vi "String Scroll.vi"(11 "fp string refnum in":refnum<vi>) -> ()   [LabVIEW 2012]
doc: "SciScan 1.2 160622"
uses:
  <vilib>/Utility/inputDevices.llb/closeMouse.vi
  <vilib>/Utility/inputDevices.llb/mouseAcquire.vi
panel:
  in  "Error In":errorcluster
  out "Error Out":errorcluster
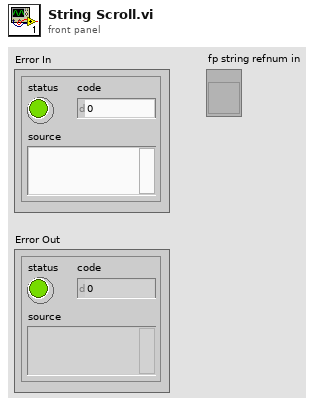
[diagram p1: front panel]
types:
  T1 = cluster{"Horizontal":i32, "Vertical":i32, "Scrolling":i32}
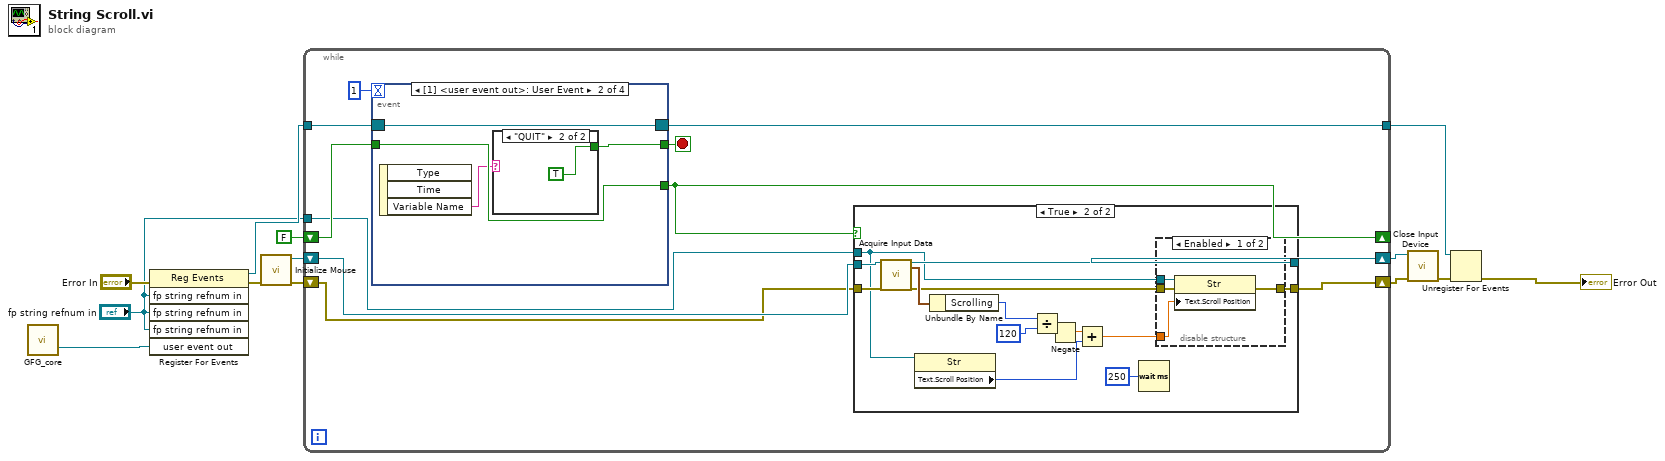
[diagram p0: block diagram]
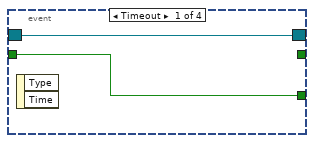
[diagram p2: hidden frame]
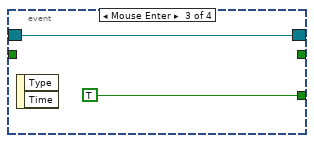
[diagram p4: hidden frame]
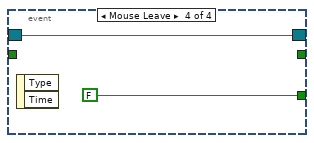
[diagram p5: hidden frame]
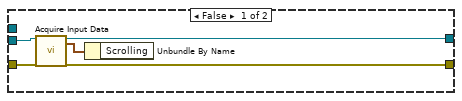
[diagram p6: hidden frame]
diagram:
  n1 = call "GFG_core.vi"() -> ("user event out"=w2:refnum<user-event>)  [unwired: 13 in, 6 out]
  n2 = register-events(error in="Error In", "fp string refnum in", "fp string refnum in", "fp string refnum in", w2) -> (reference out=w10:refnum<event-registration>, error out=w11:errorcluster)  [unwired: 1 in]
  n3 = call <vilib>:"Initialize Mouse.vi"("error in (no error)"=w11) -> ("error out"=w4:errorcluster, "device ID"=w3:refnum<k1>)  [unwired: 9 in]
  n4 = while {
    shift-right: [w21] -> w6
    shift-left: w4 -> [w23]
    shift-right: [w22] -> w5
    shift-left: w3 -> [w24]
    shift-right: [w19] -> _
    shift-left: FALSE -> [w18]
    tunnel: [w17] -> w7
    tunnel: "fp string refnum in" -> [w16]
    tunnel: w10 -> [w15]
    stop <- w14 stop-if-true
    n5 = event shown="[1] <user event out>: User Event" {
      selector: w15 -> [w25 w28 w32 w34]
      dyn-events: [w25 w28 w32 w34] -> w17
      timeout: 1 -> [_ _ _ _]
      tunnel: [w26 w29 TRUE FALSE] -> w19
      tunnel: w18 -> [w26 w29 _ _]
      tunnel: [_ w30 _ _] -> w14
      event Timeout {
        n6 = event-data() -> ()  [unwired: 1 in, 2 out]
      }
      event User Event {
        n7 = event-data() -> ("Variable Name"=w27:string)  [unwired: 1 in, 2 out]
        n8 = case shown="\"QUIT\"" w27 {
          tunnel: [_ TRUE] -> w30
          frame "False", Default {
          }
          frame "QUIT" {
          }
        }
      }
      event Mouse Enter {
        n9 = event-data() -> ()  [unwired: 1 in, 2 out]
      }
      event Mouse Leave {
        n10 = event-data() -> ()  [unwired: 1 in, 2 out]
      }
    }
    n11 = case shown="True" w19 {
      tunnel: w24 -> [w39 w54]
      tunnel: w23 -> [w40 w53]
      tunnel: [w38 w52] -> w22
      tunnel: [w37 w49] -> w21
      tunnel: w16 -> [_ w46]
      frame False {
        n12 = call-poly <vilib>:"Acquire Input Data.vi"("device ID"=w39, "error in (no error)"=w40) -> ("device ID"=w38:refnum<k1>, "axis info"=w36:T1, "error out"=w37:errorcluster)  [unwired: 14 in, 1 out]
        n13 = Unbundle By Name(w36) -> ()  [unwired: 1 out]
      }
      frame True {
        n14 = call-poly <vilib>:"Acquire Input Data.vi"("device ID"=w54, "error in (no error)"=w53) -> ("device ID"=w52:refnum<k1>, "axis info"=w51:T1, "error out"=w50:errorcluster)  [unwired: 14 in, 1 out]
        n15 = property class="Str"(reference=w46) -> ("Text.Scroll Position"=w44:u32)  [unwired: 1 in, 2 out]
        n16 = Unbundle By Name(w51) -> ("Scrolling"=w48:i32)
        n17 = Divide(x=w48, y=120) -> (x/y=w45:dbl)
        n18 = Negate(x=w45) -> (-x=w42:dbl)
        n19 = Add(x=w42, y=w44) -> (x+y=w43:dbl)
        n20 = Wait (ms)(milliseconds to wait=u32 250) -> ()  [unwired: 1 out]
        n21 = disable-structure shown="Enabled" {
          disable-tunnel: w50 -> [w58 _]
          disable-tunnel: [w57 _] -> w49
          disable-tunnel: w46 -> [w56 _]
          disable-tunnel: w43 -> [w55 _]
          frame Enabled {
            n22 = property class="Str"(reference=w56, error in=w58, "Text.Scroll Position"=w55) -> (error out=w57:errorcluster)  [unwired: 1 out]
          }
          frame Disabled {
          }
        }
      }
    }
  }
  n23 = call-poly <vilib>:"Close Input Device.vi"("error in (no error)"=w6, "device ID"=w5) -> ("error out"=w8:errorcluster)  [unwired: 8 in]
  n24 = Unregister For Events(event registration refnum=w7, error in=w8) -> (error out=→"Error Out":errorcluster)
